vi "GoTo.vi"(8 "error in (no error)":errorcluster, 10 "Robot":refnum<class "Robot.lvclass">, 11 "GoToSkill in":refnum<class "GoToSkill.lvclass">) -> (0 "error out":errorcluster, 2 "Robot out":refnum<class "Robot.lvclass">, 3 "GoToSkill out":refnum<class "GoToSkill.lvclass">)   [LabVIEW 2023, in "GoToSkill.lvclass"]
uses:
  GoToSkill.lvclass
  Robot_class/Robot.lvclass
  Robot_class/Robot.lvclass/Robot.ctl
  Robot_class/Write dest_x.vi
  Robot_class/Write dest_y.vi
  Robot_class/Write dest_orientation.vi
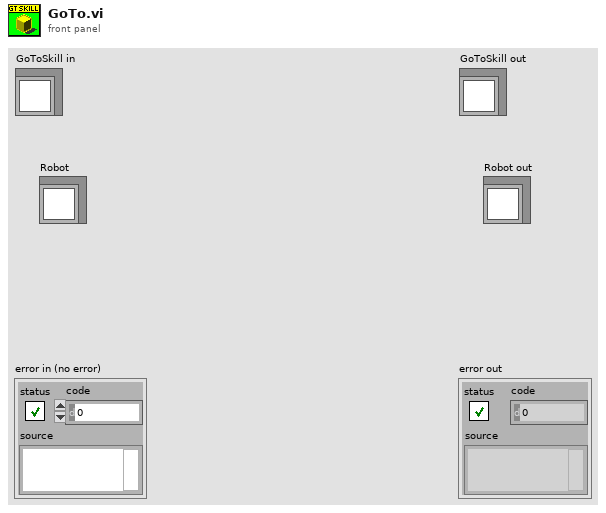
[diagram p1: front panel]
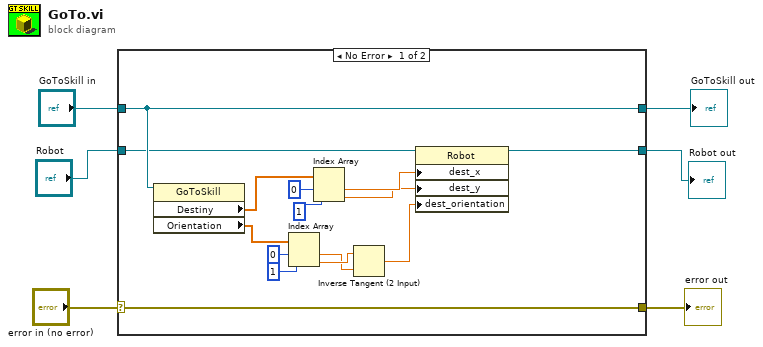
[diagram p0: block diagram]
diagram:
  n1 = case shown="No Error" "error in (no error)" {
    selector: "error in (no error)" -> [w21 w24]
    tunnel: [w21 w24] -> w5
    tunnel: [w9 w23] -> w3
    tunnel: "GoToSkill in" -> [w9 w23]
    tunnel: "Robot" -> [w8 w22]
    tunnel: [w7 w22] -> w1
    frame No Error {
      n2 = property class="GoToSkill"(reference=w9) -> ("Destiny"=w18:dbl[], "Orientation"=w15:dbl[])  [unwired: 1 in, 2 out]
      n3 = Index Array(array=w15, index #1=0 ("index"), index #2=1 ("index")) -> (element #1=w10:dbl, element #2=w11:dbl)
      n4 = Index Array(array=w18, index #1=0 ("index"), index #2=1 ("index")) -> (element #1=w17:dbl, element #2=w16:dbl)
      n5 = Inverse Tangent (2 Input)(1:w10, 2:w11) -> (0:w12:dbl)
      n6 = property class="Robot"(reference=w8, "dest_x"=w17, "dest_y"=w16, "dest_orientation"=w12) -> (reference out=w7:refnum<class "Robot.lvclass">)  [unwired: 1 in, 1 out]
    }
    frame Error {
    }
  }
  "error out" <- w5
  "GoToSkill out" <- w3
  "Robot out" <- w1
